vi "refMgr_Example2.vi"() -> ()   [LabVIEW 2017]
uses:
  <vilib>/Utility/miscctls.llb/LVPointTypeDef.ctl
  07424644-4ffc-4032-bae0-7824c00a466b.vi
  15b02cfa-01a6-4ae7-bcef-fb7d2f2e513b.vi
  5385add8-b32b-4daf-88ed-1f1d3b497987.vi
  c458119d-68f1-40af-90e0-e2bfe70ffe3d.vi
  07424644-4ffc-4032-bae0-7824c00a466b.vi/1b47866c-8e2d-43a7-815f-8cf18635e5a1.vi
  <userlib>/_NEVSTOP/TagDB/_Support/Error/_Clear Errors.vi
  15b02cfa-01a6-4ae7-bcef-fb7d2f2e513b.vi/29b2ea6d-6d7f-4e4a-ad31-a5cb760462c7.vi
  RefManager/_Support/Error/[-50011] Instance Not Found.vi
  RefManager/_Support/Error/[-50010] Mutiple Instances.vi
  5385add8-b32b-4daf-88ed-1f1d3b497987.vi/44092bd3-709c-4e20-87d5-ef7c9706681c.vi
  <userlib>/_NEVSTOP/TagDB/_Support/DataAccess/_NameCacher.vi
  07424644-4ffc-4032-bae0-7824c00a466b.vi/1b47866c-8e2d-43a7-815f-8cf18635e5a1.vi/29b2ea6d-6d7f-4e4a-ad31-a5cb760462c7.vi
  5385add8-b32b-4daf-88ed-1f1d3b497987.vi/44092bd3-709c-4e20-87d5-ef7c9706681c.vi/29b2ea6d-6d7f-4e4a-ad31-a5cb760462c7.vi
  <userlib>/_NEVSTOP/TagDB/_Support/Change Detector/TagDB dbChanged.vi
  <userlib>/_NEVSTOP/TagDB/_Support/DataAccess/TagDB Ref to DVR.vi
  <userlib>/_NEVSTOP/TagDB/_Support/Error/_[error50000]Invalid DB REF.vi
  <userlib>/_NEVSTOP/TagDB/_Support/URL/TRIM-BOTH-SPACE.vi
  <userlib>/_NEVSTOP/TagDB/_Support/Error/_[error50002]Invalid DataType.vi
  <userlib>/_NEVSTOP/TagDB/_Support/Error/_Build Error Cluster.vi
  RefManager/TagDB RefManager.lvlib
  <userlib>/_NEVSTOP/TagDB/TagDB.lvlib
panel:
  in  "Key":string="Array"
  in  "Reset":bool
  out "::Origin::":T1
  out "::DB items::":string[](array[string])
  out "::DataChangeFlag::":timestamp
  out "::DataItemFlag::":timestamp
  in  "Tab Control":enum32{"Page 1", "Page 2", "Page 3"}(tab)
  out "Waveform Chart 2":dbl(graph)
  out "Waveform Chart 3":dbl(graph)
  in  "Tab Control 2":enum32{"Page 1", "Page 2", "Page 3"}(tab)
  out "Waveform Chart 4":dbl(graph)
  out "Waveform Chart 5":dbl(graph)
  out "Waveform Chart 1":dbl(graph)
  in  "Combo Box":string(combo)
  out "VI Name":string
  out "Cluster":errorcluster
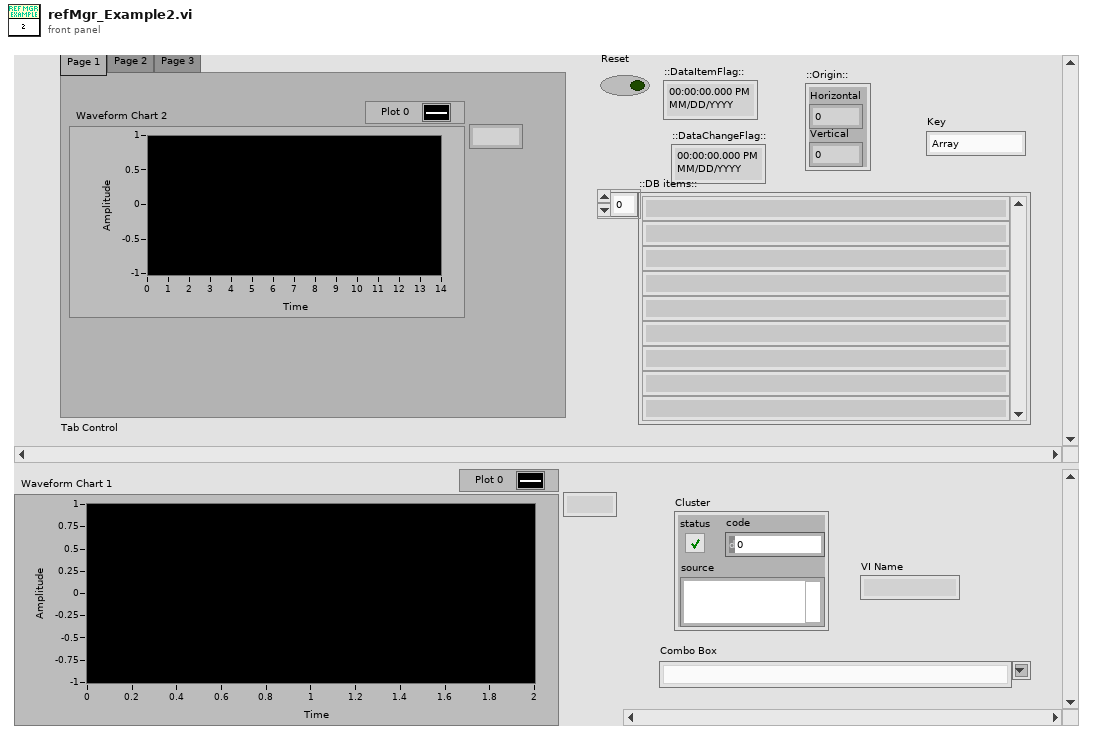
[diagram p1: front panel]
types:
  T1 = typedef "LVPointTypeDef.ctl" = cluster{"Horizontal":i16, "Vertical":i16}
  T2 = typedef "TagDB.lvlib/TagDB.ctl" = refnum<k1>
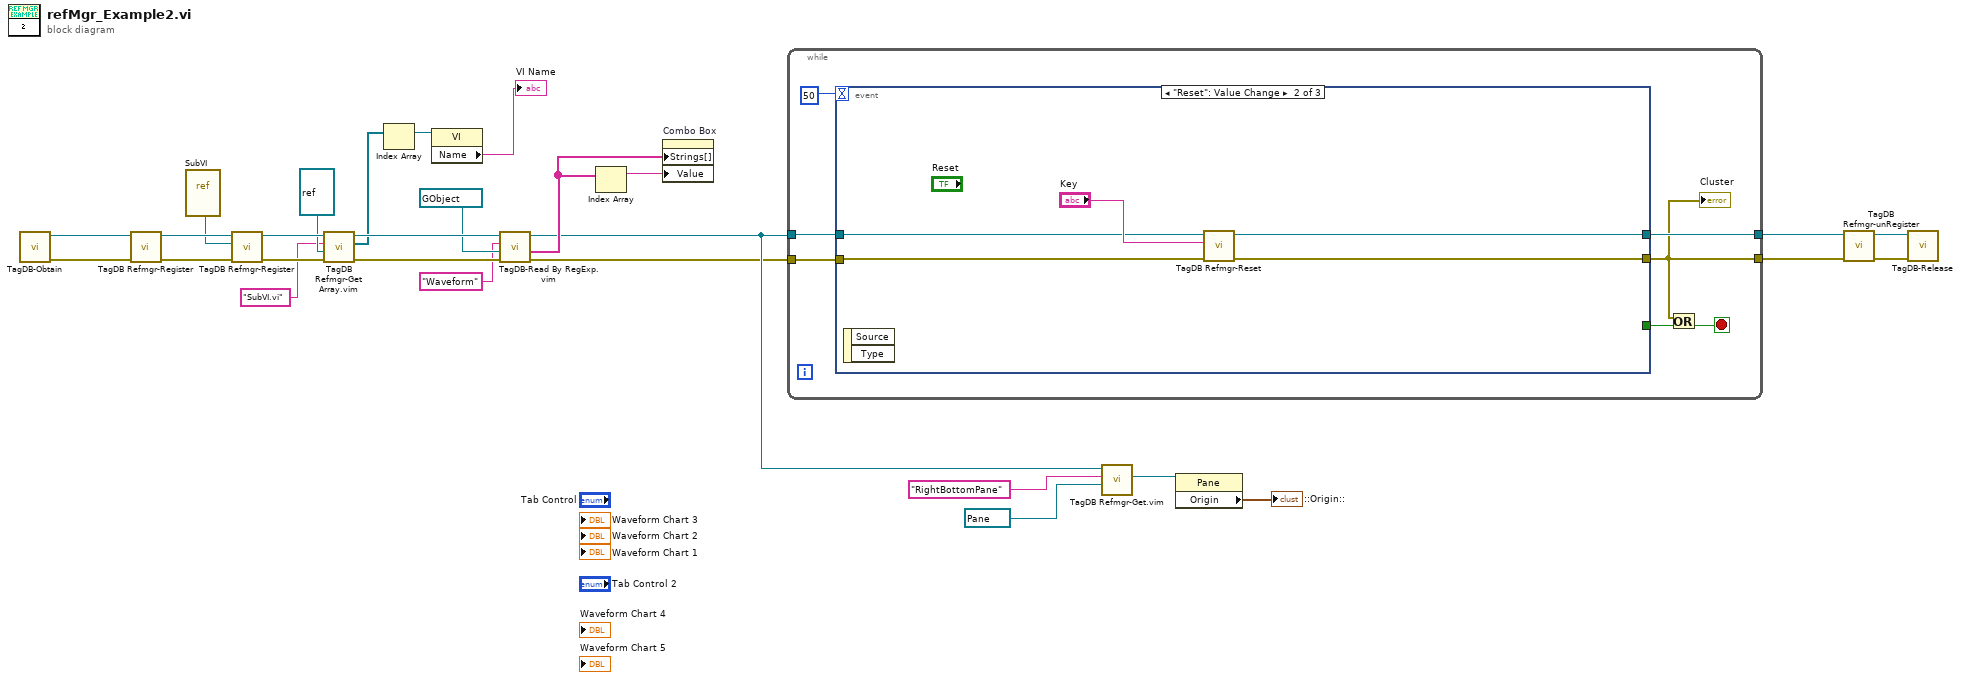
[diagram p0: block diagram]
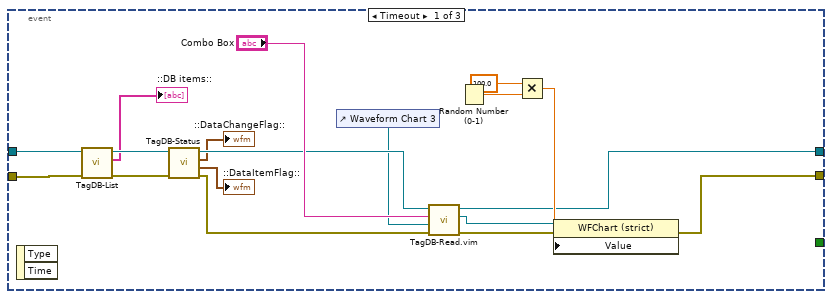
[diagram p2: hidden frame]
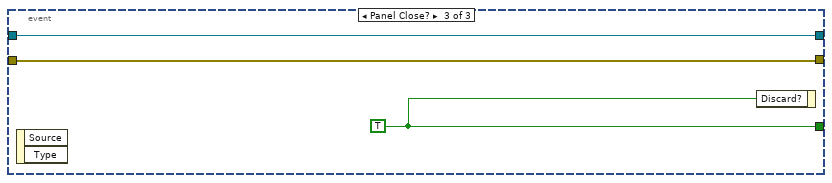
[diagram p3: hidden frame]
diagram:
  n1 = call <userlib>:"TagDB-Obtain.vi"() -> ("error out"=w26:errorcluster, "TagDB"=w27:T2)  [unwired: 5 in, 1 out]
  n2 = call "TagDB Refmgr-Register.vi"("error in (no error)"=w26, "TagDB in"=w27) -> ("error out"=w24:errorcluster, "TagDB out"=w25:T2)  [unwired: 7 in, 1 out]
  n3 = vi-ref "SubVI.vi"() -> (w23:refnum<vi>)
  n4 = call "TagDB Refmgr-Register.vi"("error in (no error)"=w24, "VI Refnum"=w23, "TagDB in"=w25) -> ("error out"=w16:errorcluster, "TagDB out"=w17:T2)  [unwired: 6 in, 1 out]
  n5 = call "TagDB Refmgr-Get Array.vim"("error in (no error)"=w16, "Type"=refnum<vi> refnum ("reference out"), "RegExp"="SubVI.vi" ("Key"), "DB Ref"=w17) -> ("error out"=w14:errorcluster, "References"=w1:refnum<vi>[], "DB Ref(dup)"=w15:T2)  [unwired: 4 in, 1 out]
  n6 = Index Array(array=w1) -> (element=w8:refnum<vi>)  [unwired: 1 in]
  n7 = property class="VI"(reference=w8) -> ("Name"=→"VI Name":string)  [unwired: 1 in, 2 out]
  n8 = call "TagDB-Read By RegExp.vim"("error in (no error)"=w14, "Type"=refnum<vi> refnum, "RegExp"="Waveform" ("Pattern"), "DB Ref"=w15) -> ("error out"=w2:errorcluster, "names"=w7:string[], "DB Ref(dup)"=w3:T2)  [unwired: 4 in, 1 out]
  n9 = Index Array(array=w7) -> (element=w28:string)  [unwired: 1 in]
  n10 = property on="Combo Box" class="CmbBox"("Strings[]"=w7, "Value"=w28) -> ()  [unwired: 2 in, 2 out]
  n11 = while {
    tunnel: w3 -> [w33]
    tunnel: w2 -> [w32]
    tunnel: [w31] -> w22
    tunnel: [w29] -> w20
    stop <- w30 stop-if-true
    n12 = event shown="[1] \"Reset\": Value Change" {
      selector: _ -> [_ _ _]
      dyn-events: _ -> [_ _ _]
      timeout: u32 50 ("milliseconds to wait") -> [_ _ _]
      tunnel: [_ _ w61] -> w35
      tunnel: w33 -> [w46 w57 w60]
      tunnel: w32 -> [w38 w56 w59]
      tunnel: [w40 w54 w60] -> w31
      tunnel: [w47 w55 w59] -> w29
      event Timeout {
        n13 = event-data() -> ()  [unwired: 1 in, 2 out]
        n14 = call <userlib>:"TagDB-List.vi"("error in (no error)"=w38, "TagDB"=w46) -> ("error out"=w37:errorcluster, "names"=→"::DB items::":string[], "TagDB(dup)"=w45:T2)  [unwired: 6 in, 1 out]
        n15 = call <userlib>:"TagDB-Status.vi"("error in (no error)"=w37, "DB Ref"=w45) -> ("error out"=w43:errorcluster, "Item Change Timestamp"=→"::DataItemFlag::":timestamp, "Global Change Timestamp"=→"::DataChangeFlag::":timestamp, "DB Ref(dup)"=w44:T2)  [unwired: 4 in, 2 out]
        n16 = control-ref of="Waveform Chart 3"() -> (w36:refnum<vi>)
        n17 = call "TagDB-Read.vim"("error in (no error)"=w43, "Type(empty to read as variant)"=w36, "name"="Combo Box", "TagDB"=w44) -> ("error out"=w52:errorcluster, "Value"=w53:refnum<vi>, "TagDB(dup)"=w40:T2)  [unwired: 2 in, 3 out]
        n18 = Random Number (0-1)() -> (number: 0 to 1=w49:dbl)
        n19 = Multiply(x=100.0, y=w49) -> (x*y=w51:dbl)
        n20 = property class="WFChart (strict)"(reference=w53, error in=w52, "Value"=w51) -> (error out=w47:errorcluster)  [unwired: 1 out]
      }
      event "Reset": Value Change {
        n21 = event-data() -> ()  [unwired: 1 in, 2 out]
        n22 = call "TagDB Refmgr-Reset.vi"("error in (no error)"=w56, "RegExp"="Key", "TagDB in"=w57) -> ("error out"=w55:errorcluster, "TagDB out"=w54:T2)  [unwired: 6 in, 1 out]
      }
      event Panel Close? {
        w61 = TRUE
        n23 = event-data() -> ()  [unwired: 1 in, 2 out]
        n24 = event-data("Discard?"=w61) -> ()  [unwired: 1 in, 1 out]
      }
    }
    "Cluster" <- w29
    n25 = Or(x=w29, y=w35) -> (x .or. y?=w30:bool)
  }
  n26 = call "TagDB Refmgr-Get.vim"("Type"=refnum<vi> refnum ("Reference"), "RegExp"="RightBottomPane" ("Key"), "DB Ref"=w3) -> ("Reference"=w4:refnum<vi>)  [unwired: 5 in, 3 out]
  n27 = property class="Pane"(reference=w4) -> ("Origin"=→"::Origin::":T1)  [unwired: 1 in, 2 out]
  n28 = call "TagDB Refmgr-unRegister.vi"("error in (no error)"=w20, "TagDB in"=w22) -> ("error out"=w19:errorcluster, "TagDB out"=w21:T2)  [unwired: 8 in]
  n29 = call <userlib>:"TagDB-Release.vi"("error in (no error)"=w19, "TagDB"=w21) -> ()  [unwired: 9 in, 1 out]
